vi "Playground.vi"() -> ()   [LabVIEW 2019]
uses:
  ObjectSettings/ObjectSettings.lvclass/ObjectSettings.ctl
  Setting Database/Setting Database.lvclass
  <vilib>/JKI/JKI SMO/SMO/SMO.lvclass
  Path Settings/Path Settings.lvclass
  C:/Users/Albro/Documents/GitHub/AFM-Lithography/lvsrc/Classes/Settings/ObjectSettings/ObjectSettings.lvclass
  Setting Database/Typedefs/PrivateEvents--Setting Database.CopyActivePathToAll.ctl
  <vilib>/addons/_JKI Toolkits/Caraya/classes/Test/Test.lvclass
  <vilib>/addons/_JKI Toolkits/Caraya/classes/Assert/Assert.lvclass
  <vilib>/addons/_JKI Toolkits/Caraya/classes/Assert/Assert Equal Value_Variant.vi
  ObjectSettings/ObjectSettings.lvclass
  C:/Program Files (x86)/National Instruments/LabVIEW 2019/vi.lib/JKI/JKI SMO/SMO/SMO.lvclass
  Setting Database/Typedefs/PrivateEvents--Setting Database.Refresh.ctl
panel:
  in  "Speed Settings":bool
  out "error out":errorcluster
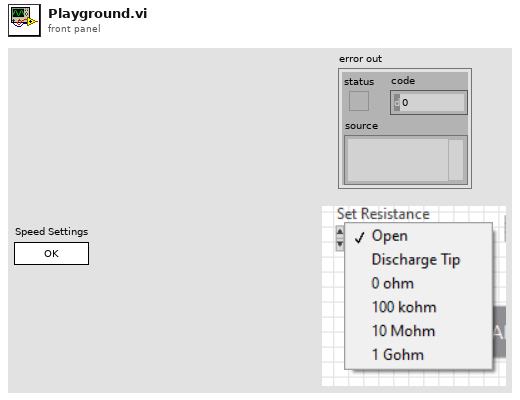
[diagram p1: front panel]
types:
  T1 = typedef "Setting Database.lvclass/PrivateEvents--Setting Database.Refresh.ctl" = cluster{"Paths":string[], "Rectangles":string[], "Funnels":string[], "Dots":string[]}
  T2 = typedef "Setting Database.lvclass/PublicEvents--Cluster.ctl" = cluster{"NewActivePath":refnum<user-event>, "PathsUpdated":refnum<user-event>, "RectanglesUpdated":refnum<user-event>, "NewActiveRectangle":refnum<user-event>, "NewActiveFunnel":refnum<user-event>, "FunnelsUpdated":refnum<user-event>, "NewActiveDot":refnum<user-event>, "DotsUpdated":refnum<user-event>}
  T3 = typedef "Setting Database.lvclass/PublicEvents--Setting Database.PathsUpdated.ctl" = refnum<class "Path Settings.lvclass">[]
  T4 = enum32{"Invalid", "Standard", "Closed", "Hidden", "Minimized", "Maximized"}
  T5 = enum32{"invalid app kind", "Development System", "Run Time System", "Student Edition", "Embedded LabVIEW", "Evaluation", "Custom"}
  T6 = typedef "Setting Database.lvclass/PrivateEvents--Setting Database.CopyActivePathToAll.ctl" = bool
  T7 = typedef "Setting Database.lvclass/PublicEvents--Setting Database.NewActivePath.ctl" = refnum<class "Path Settings.lvclass">
  T8 = cluster{"Core":cluster{"Current VI Reference":refnum<vi>, "Close Panel on Exit?":bool}, "Path Settings":refnum<class "Path Settings.lvclass">, "Your string data":string, "Setting Database":refnum<class "Setting Database.lvclass">}
  T9 = cluster{"Current VI Reference":refnum<vi>, "Close Panel on Exit?":bool}
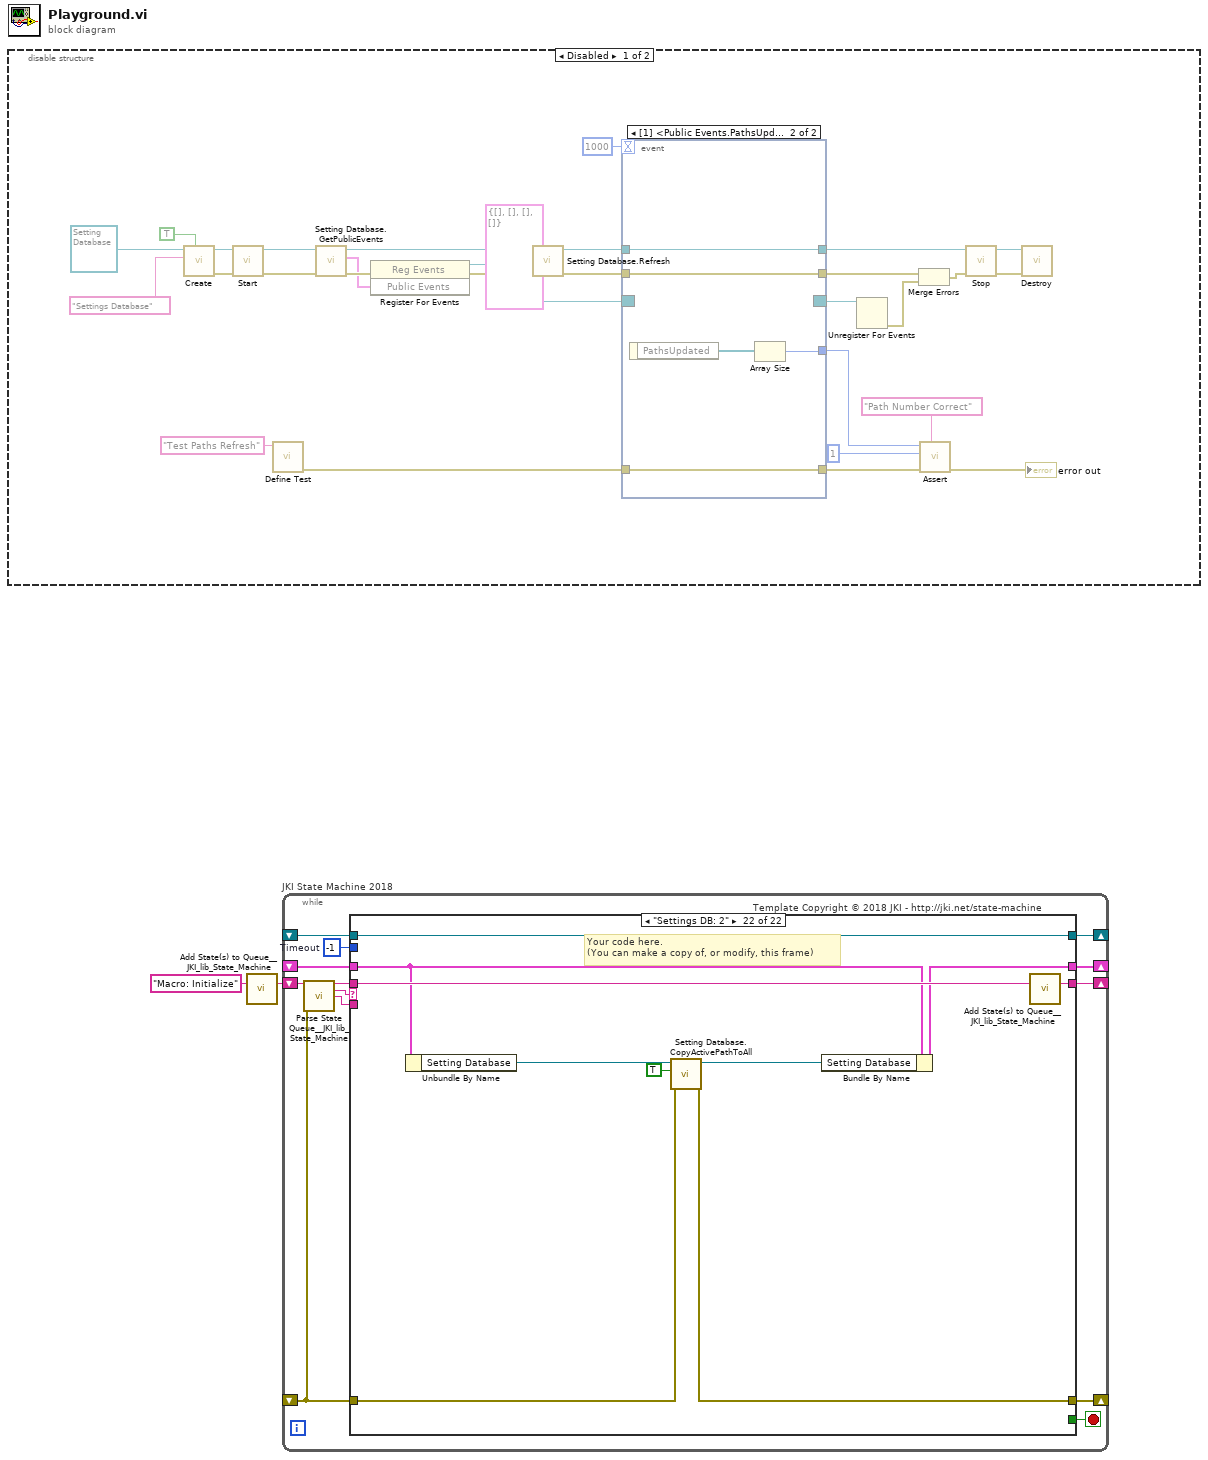
[diagram p0: block diagram]
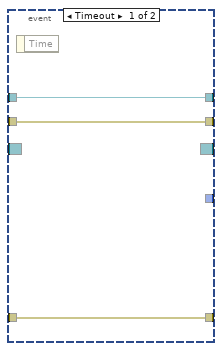
[diagram p2: hidden frame]
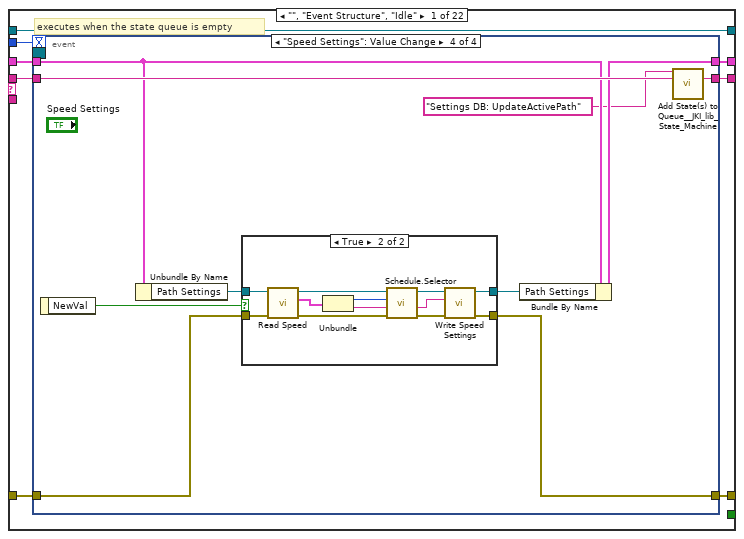
[diagram p4: hidden frame]
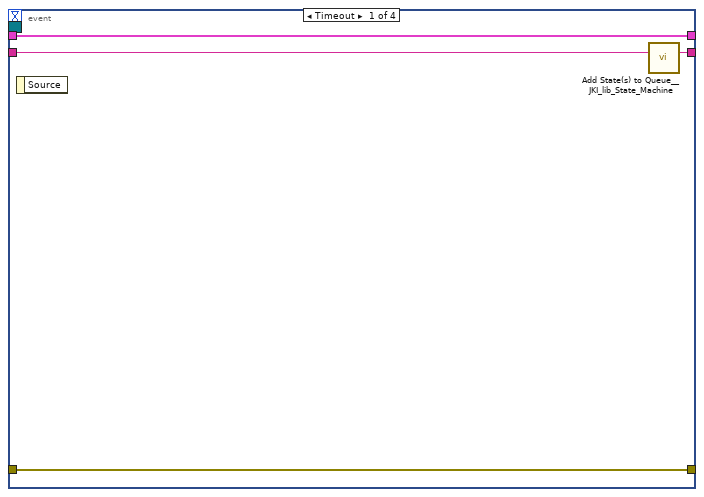
[diagram p5: hidden frame]
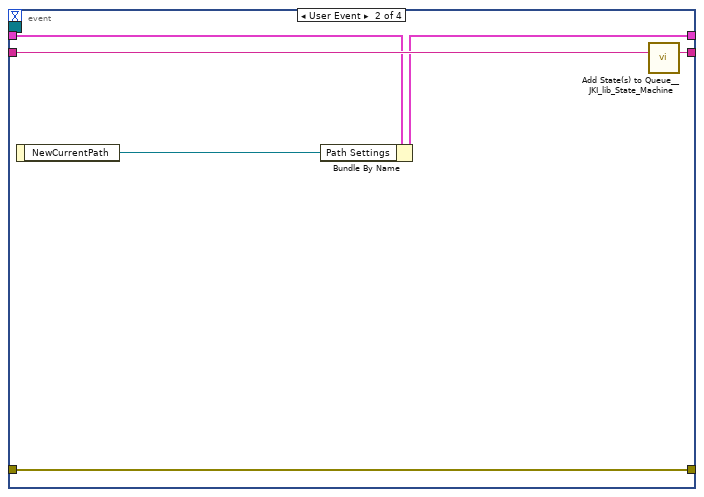
[diagram p6: hidden frame]
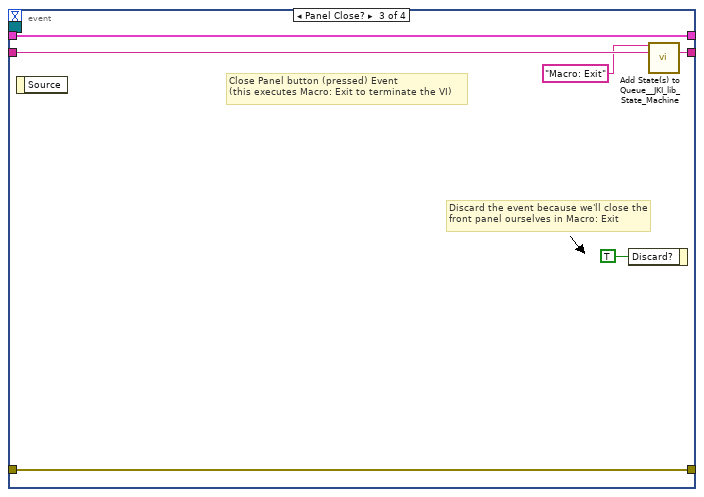
[diagram p7: hidden frame]
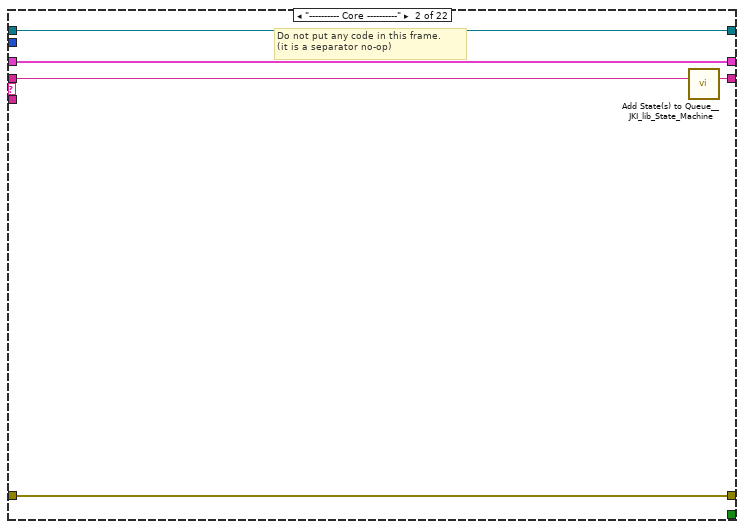
[diagram p9: hidden frame]
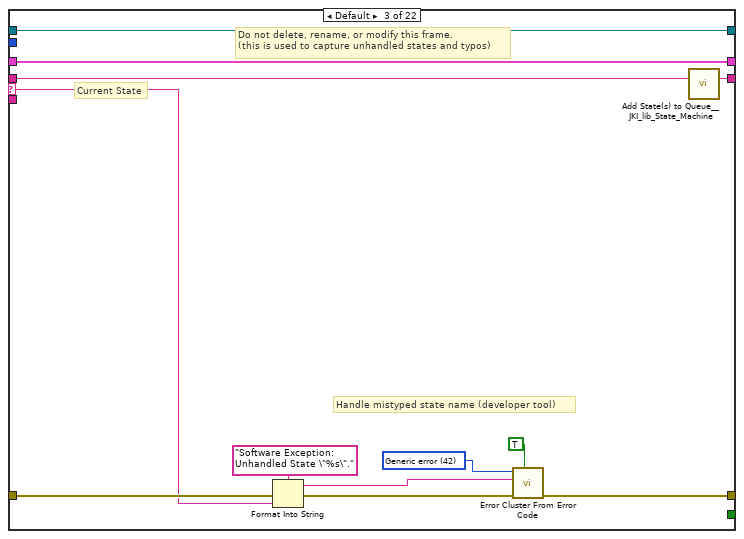
[diagram p10: hidden frame]
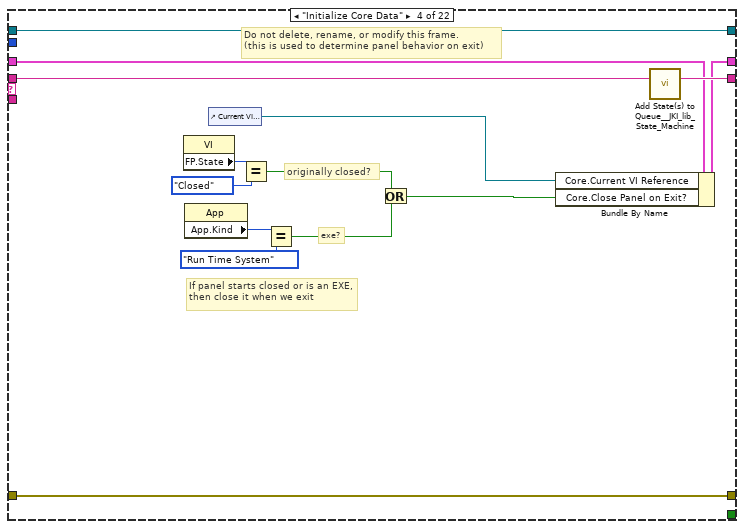
[diagram p11: hidden frame]
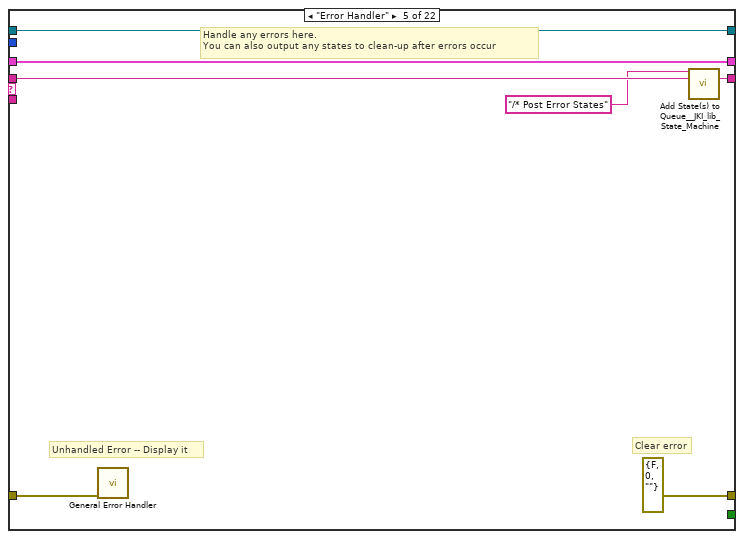
[diagram p12: hidden frame]
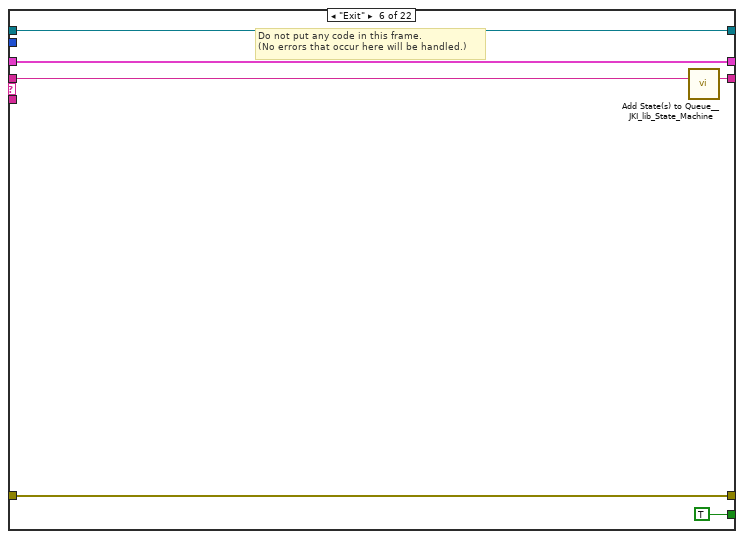
[diagram p13: hidden frame]
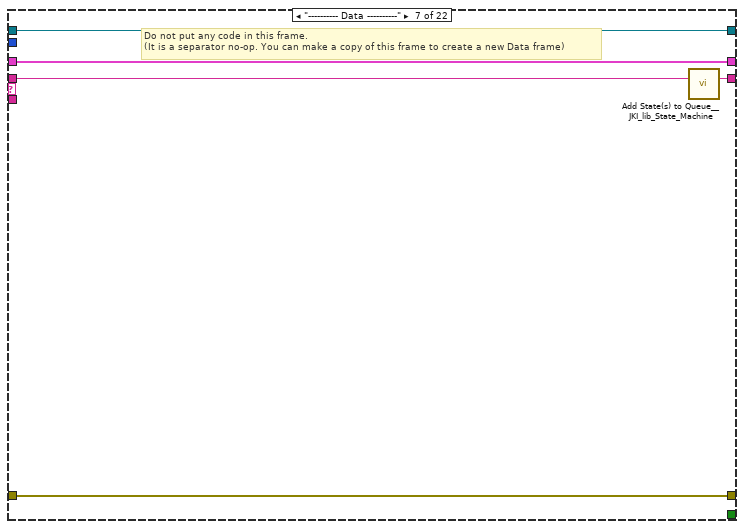
[diagram p14: hidden frame]
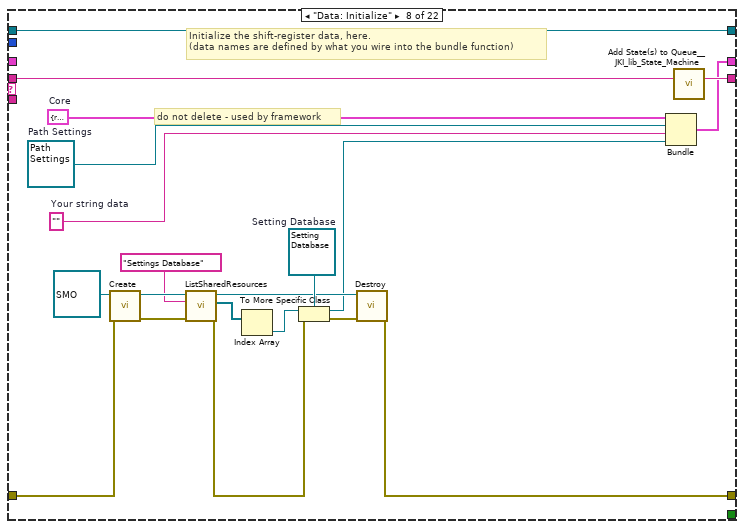
[diagram p15: hidden frame]
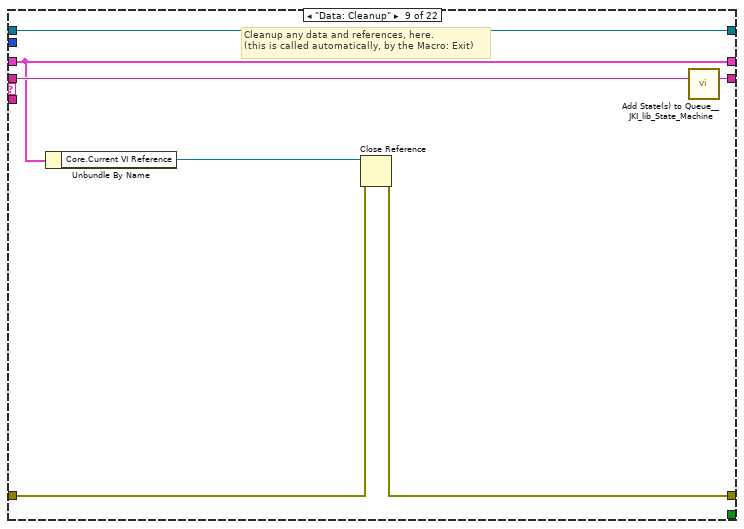
[diagram p16: hidden frame]
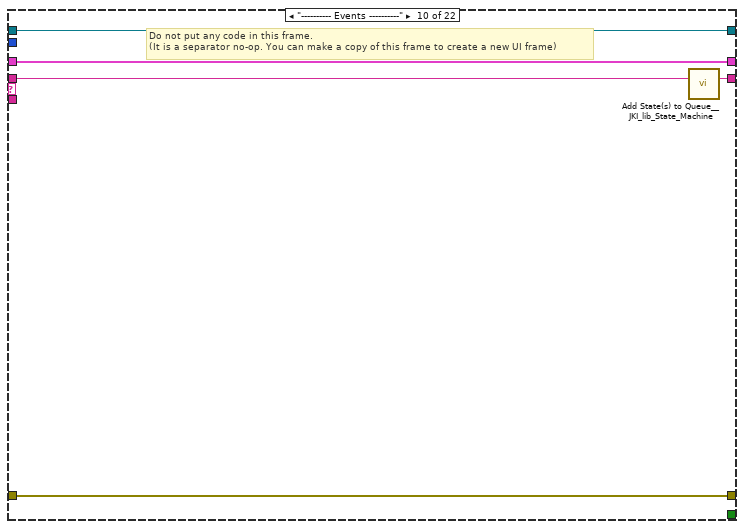
[diagram p17: hidden frame]
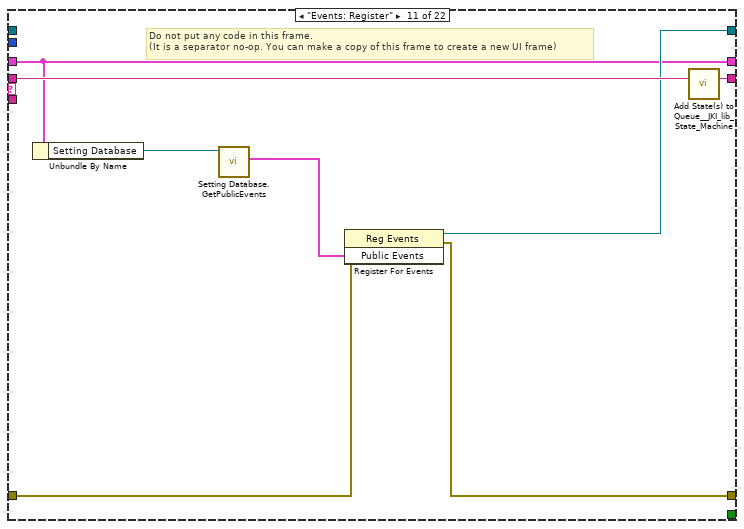
[diagram p18: hidden frame]
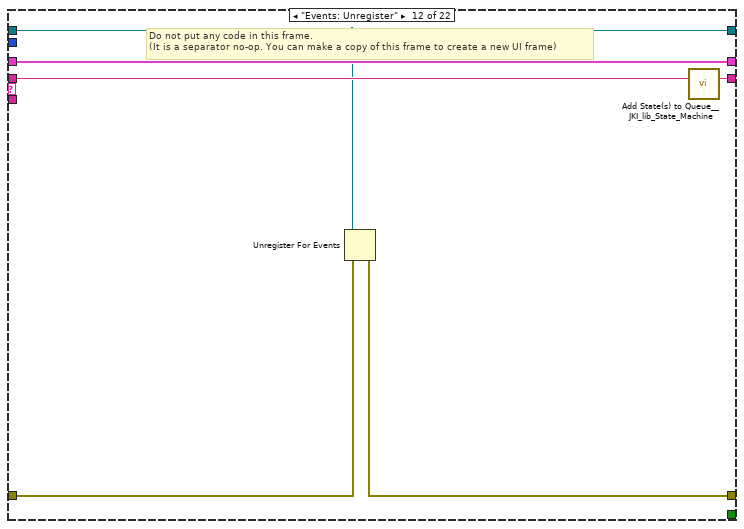
[diagram p19: hidden frame]
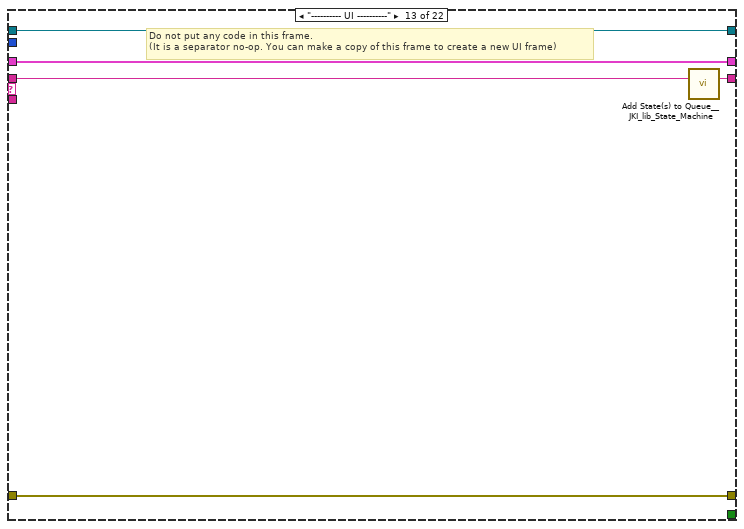
[diagram p20: hidden frame]
diagram:
  n1 = disable-structure shown="Disabled" {
    frame Disabled {
      n2 = call <vilib>:"Create.vi"("Shared Resource (F)"=TRUE, "Subsystem Name (optional)"="Settings Database", "SMO"=refnum<class "Setting Database.lvclass"> refnum ("Setting Database.lvclass")) -> ("error out"=w4:errorcluster, "SMO out"=w29:refnum<class "Setting Database.lvclass">)  [unwired: 6 in, 1 out]
      n3 = call <vilib>:"Start.vi"("error in (no error)"=w4, "SMO"=w29) -> ("error out"=w27:errorcluster, "SMO out"=w26:refnum<class "Setting Database.lvclass">)  [unwired: 8 in]
      n4 = call <vilib>:"Define Test.vi"("Label (VI Title)"="Test Paths Refresh") -> ("error out"=w11:errorcluster)  [unwired: 9 in, 1 out]
      n5 = call "Setting Database.GetPublicEvents.vi"("error in (no error)"=w27, "Setting Database"=w26) -> ("error out"=w24:errorcluster, "Public Events"=w22:T2, "Setting Database out"=w25:refnum<class "Setting Database.lvclass">)  [unwired: 7 in]
      n6 = register-events(error in=w24, w22) -> (reference out=w3:refnum<event-registration>, error out=w23:errorcluster)  [unwired: 1 in]
      n7 = call "Setting Database.Refresh.vi"("error in (no error)"=w23, "Initialize"=T1 {"Paths"=[], "Rectangles"=[], "Funnels"=[], "Dots"=[]}, "Setting Database"=w25) -> ("error out"=w17:errorcluster, "Setting Database out"=w18:refnum<class "Setting Database.lvclass">)  [unwired: 7 in]
      n8 = event shown="[1] <Public Events.PathsUpdated>: User Event" {
        selector: w3 -> [_ _]
        dyn-events: [_ _] -> w20
        timeout: 1000 -> [_ _]
        tunnel: [w35 w40] -> w19
        tunnel: w18 -> [w35 w40]
        tunnel: w17 -> [w34 w39]
        tunnel: [w34 w39] -> w16
        tunnel: [_ w37] -> w7
        tunnel: w11 -> [w33 w36]
        tunnel: [w33 w36] -> w10
        event Timeout {
          n9 = event-data() -> ()  [unwired: 1 in, 1 out]
        }
        event User Event {
          n10 = event-data() -> ("PathsUpdated"=w38:T3)  [unwired: 1 in]
          n11 = Array Size(array=w38) -> (size(s)=w37:i32)
        }
      }
      n12 = Unregister For Events(event registration refnum=w20) -> (error out=w14:errorcluster)  [unwired: 1 in]
      n13 = Merge Errors(w16, w14) -> (w15:errorcluster)
      n14 = call-poly <vilib>:"Assert.vi"("Label"="Path Number Correct", "error in (no error)"=w10, "Actual"=1 ("size(s)"), "Expected"=w7) -> ("error out"=→"error out":errorcluster)  [unwired: 6 in, 1 out]
      n15 = call <vilib>:"Stop.vi"("error in (no error)"=w15, "SMO"=w19) -> ("error out"=w13:errorcluster, "SMO out"=w28:refnum<class "Setting Database.lvclass">)  [unwired: 8 in]
      n16 = call <vilib>:"Destroy.vi"("error in (no error)"=w13, "SMO"=w28) -> ()  [unwired: 9 in, 1 out]
    }
    frame Enabled {
    }
  }
  n17 = call <vilib>:"Add State(s) to Queue__JKI_lib_State_Machine.vi"("State(s) in (\"\")"="Macro: Initialize") -> ("States Out"=w2:string)  [unwired: 14 in]
  n18 = while "JKI State Machine 2018" {
    shift-right: [w46] -> _
    shift-left: _ -> [w45]
    shift-right: [w49] -> _
    shift-left: _ -> [w43]
    shift-right: [w48] -> _
    shift-left: w2 -> [w50]
    shift-right: [w42] -> _
    shift-left: _ -> [w41]
    stop <- w47 stop-if-true
    w44 = -1  # Timeout
    # "Template Copyright © 2018 JKI - http://jki.net/state-machine"
    n19 = call <vilib>:"Parse State Queue__JKI_lib_State_Machine.vi"("State Queue"=w50, "Error In (no error)"=w43) -> ("Remaining States"=w52:string, "Current State"=w53:string, "Arguments"=w51:string)  [unwired: 11 in]
    n20 = case shown="\"Settings DB: 2\"" w53 {
      selector: w53 -> [_ _ w108 _ _ _ _ _ _ _ _ _ _ _ _ _ _ _ _ _ _ _]
      tunnel: w52 -> [w61 w106 w112 w132 w139 w145 w150 w170 w177 w182 w190 w196 w201 w206 w213 w225 w295 w301 w312 w317 w327 w337]
      tunnel: w51 -> [_ _ _ _ _ _ _ _ _ _ _ _ _ _ w208 w219 _ _ _ _ _ _]
      tunnel: w45 -> [w59 w103 w110 w125 w136 w143 w147 _ w172 w179 w186 w194 w198 w204 w211 w221 w292 w298 w309 w314 w324 w328]
      tunnel: [w58 w104 w114 w129 errorcluster {"status"=FALSE, "code"=0, "source"=""} ("error out") w142 w148 w153 w173 w180 w187 w191 w199 w203 w209 w222 w293 w299 w310 w315 w320 w334] -> w49
      tunnel: w43 -> [w57 w104 w113 w129 w135 w142 w148 w155 w174 w180 w183 w192 w199 w203 w210 w223 w293 w299 w310 w315 w319 w333]
      tunnel: [w60 w105 w111 w131 w138 w144 w149 w169 w176 w181 w189 w195 w200 w205 w212 w224 w294 w300 w311 w316 w326 w336] -> w48
      tunnel: [_ _ _ _ _ TRUE _ _ _ _ _ _ _ _ _ _ _ _ _ _ _ _] -> w47
      tunnel: [w56 w103 w110 w130 w136 w143 w147 w168 w172 w179 w186 w194 w198 w204 w211 w221 w292 w298 w309 w314 w325 w329] -> w46
      tunnel: w44 -> [w55 _ _ _ _ _ _ _ _ _ _ _ _ _ _ _ _ _ _ _ _ _]
      tunnel: [w54 w102 w107 w119 w133 w140 w146 w151 w171 w178 w188 w193 w197 w202 w207 w218 w291 w296 w302 w313 w318 w335] -> w42
      tunnel: w41 -> [w54 w102 w107 w119 w133 w140 w146 w151 w171 w178 _ w193 w197 w202 w207 w218 w291 w296 w302 w313 w318 w335]
      frame "", "Event Structure", "Idle" {
        # "executes when the state queue is empty"
        n21 = event shown="[3] \"Speed Settings\": Value Change" {
          selector: w54 -> [_ _ _ _]
          dyn-events: _ -> [_ _ _ _]
          timeout: w55 -> [_ _ _ _]
          tunnel: w61 -> [w65 w71 w77 w87]
          tunnel: [w64 w70 w76 w86] -> w60
          tunnel: w59 -> [w62 w67 w74 w79]
          tunnel: [w63 w69 w75 w80] -> w58
          tunnel: w57 -> [w63 w69 w75 w85]
          tunnel: [w62 w68 w74 w82] -> w56
          event Timeout {
            n22 = event-data() -> ()  [unwired: 1 in, 1 out]
            n23 = call <vilib>:"Add State(s) to Queue__JKI_lib_State_Machine.vi"("State(s) in (\"\")"=w65) -> ("States Out"=w64:string)  [unwired: 14 in]
          }
          event User Event {
            n24 = event-data() -> ("NewCurrentPath"=w66:T7)  [unwired: 1 in]
            n25 = Bundle By Name(cluster=w67, "Path Settings"=w66) -> (w68:T8)
            n26 = call <vilib>:"Add State(s) to Queue__JKI_lib_State_Machine.vi"("State(s) in (\"\")"=w71) -> ("States Out"=w70:string)  [unwired: 14 in]
          }
          event Panel Close? {
            # "Discard the event because we'll close the front panel ourselves in Macro: Exit"
            # "Close Panel button (pressed) Event\n(this executes Macro: Exit to terminate the VI)"
            n27 = event-data() -> ()  [unwired: 1 in, 1 out]
            n28 = event-data("Discard?"=TRUE) -> ()  [unwired: 1 in, 1 out]
            n29 = call <vilib>:"Add State(s) to Queue__JKI_lib_State_Machine.vi"("State(s) in Front (\"\")"="Macro: Exit", "State(s) in (\"\")"=w77) -> ("States Out"=w76:string)  [unwired: 13 in]
          }
          event "Speed Settings": Value Change {
            n30 = event-data() -> ("NewVal"=w81:bool)  [unwired: 1 in]
            n31 = Unbundle By Name(w79) -> ("Path Settings"=w84:refnum<class "Path Settings.lvclass">)
            n32 = case shown="True" w81 {
              tunnel: w84 -> [w89 w94]
              tunnel: [w89 w92] -> w83
              tunnel: w85 -> [w88 w91]
              tunnel: [w88 w90] -> w80
              frame False {
              }
              frame True {
                n33 = call "Read Speed.vi"("error in (no error)"=w91, "ObjectSettings in"=w94) -> ("error out"=w97:errorcluster, "Speed"=w98:cluster{"Schedule":u16, "Settings":string}, "ObjectSettings out"=w101:refnum<class "Path Settings.lvclass">)  [unwired: 7 in]
                n34 = Unbundle(w98) -> ("Schedule"=w100:u16, "Settings"=w99:string)
                n35 = call-dynamic "Schedule.Selector.vi"("error in (no error)"=w97, "Settings In"=w99, "Schedule"=w100, "ObjectSettings in"=w101) -> ("error out"=w95:errorcluster, "Settings Out"=w93:string, "ObjectSettings out"=w96:refnum<class "Path Settings.lvclass">)  [unwired: 5 in]
                n36 = call "Write Speed Settings.vi"("error in (no error)"=w95, "Settings"=w93, "ObjectSettings in"=w96) -> ("error out"=w90:errorcluster, "ObjectSettings out"=w92:refnum<class "Path Settings.lvclass">)  [unwired: 7 in]
              }
            }
            n37 = Bundle By Name(cluster=w79, "Path Settings"=w83) -> (w82:T8)
            n38 = call <vilib>:"Add State(s) to Queue__JKI_lib_State_Machine.vi"("State(s) in Front (\"\")"="Settings DB: UpdateActivePath", "State(s) in (\"\")"=w87) -> ("States Out"=w86:string)  [unwired: 13 in]
          }
        }
      }
      frame "---------- Core ----------" {
        # "Do not put any code in this frame.\n(it is a separator no-op)"
        n39 = call <vilib>:"Add State(s) to Queue__JKI_lib_State_Machine.vi"("State(s) in (\"\")"=w106) -> ("States Out"=w105:string)  [unwired: 14 in]
      }
      frame Default {
        w117 = 42 items=["No error", "Argument error", "Memory is full", "Out of zone", "End of file", "File already open", "Generic file I/O error", "File not found", "File permission error", "Disk is full", "Duplicate path", "Too many files open", "System feature not enabled", "Resource file not found", "Cannot add resource", "Resource not found", "Image not found", "Image memory error", "Pen does not exist", "Config type invalid", "Config token not found", "Config parse error", "Config memory error", "Bad external code format", "Bad external code offset", "External code not present", "Null window", "Destroy window error", "Null menu", "Print aborted", "Bad print record", "Print driver error", "Windows error during printing", "Memory error during printing", "Print dialog error", "Generic print error", "Invalid device refnum", "Device not found", "Device parameter error", "Device unit error", "Cannot open device", "Device call aborted", "Generic error", "Cancelled by user", "Object ID too low", "Object ID too high", "Object not in heap", "Unknown heap", "Unknown object (invalid DefProc)", "Unknown object (DefProc not in table)", "Message out of range", "Invalid (null) method", "Unknown message", "Manager call not supported", "Bad address", "Network operation in progress", "Network operation timed out", "Connection is busy", "Network attribute not supported", "Network error", "Address in use", "System out of memory", "Connection aborted", "Connection refused", "Not connected", "Already connected", "Connection closed", "Initialization error (interapplication manager)", "Bad occurrence", "Wait on unbound occurrence handler", "Occurrence queue overflow", "Datalog type conflict", "Unused", "Unrecognized type (interapplication manager)", "Memory corrupt", "Failed to make temporary DLL", "Old CIN version", "Drag socket not found", "Failed to load drop-object", "Failed to register OLE object", "Failed to release OLE object", "Format specifier type mismatch", "Unknown format specifier", "Too few format specifiers", "Too many format specifiers", "Scan failed", "Newer CIN version", "Error converting to variant", "Runtime menu error", "Password tampered", "Variant attribute not found", "Incompatible variant data type", "Event data is not available", "Event Store is not present", "Occurrence is not found", "Event Queue is not created", "Event info is not available", "Refnum passed is NULL", "Error retrieving Class GUID", "Error retrieving CoClass GUID", "Error retrieving TypeLib GUID.", "Bad built application magic bytes.", "Specific driver is different from the specific driver associated with the Logical Name.", "There is no session opened to the class driver.", "Max Error", "MAX - Error with config objects", "MAX - Error loading configuration", "MAX - Group not supported"]
        # "Current State"
        # "Do not delete, rename, or modify this frame.\n(this is used to capture unhandled states and typos)"
        # "Handle mistyped state name (developer tool)"
        n40 = Format Into String(format string="Software Exception: Unhandled State \"%s\"." ("message"), error in=w113, w108) -> (resulting string=w116:string, error out=w115:errorcluster)  [unwired: 1 in]
        n41 = call <vilib>:"Error Cluster From Error Code.vi"("show call chain? (False)"=TRUE, "error in (no error)"=w115, "error message (\"\")"=w116, "error code (0)"=w117) -> ("error out"=w114:errorcluster)  [unwired: 5 in]
        n42 = call <vilib>:"Add State(s) to Queue__JKI_lib_State_Machine.vi"("State(s) in (\"\")"=w112) -> ("States Out"=w111:string)  [unwired: 14 in]
      }
      frame "Initialize Core Data" {
        # "Do not delete, rename, or modify this frame.\n(this is used to determine panel behavior on exit)"
        # "originally closed?"
        # "exe?"
        # "If panel starts closed or is an EXE, then close it when we exit"
        n43 = property class="VI"() -> ("FP.State"=w122:T4)  [unwired: 2 in, 2 out]
        n44 = property class="App"() -> ("App.Kind"=w128:T5)  [unwired: 2 in, 2 out]
        n45 = control-ref of="Current VI Reference"() -> (w123:refnum<vi>)
        n46 = Equal?(x=w122, y=T4."Closed" ("Front Panel Window:State")) -> (x = y?=w120:bool)
        n47 = Equal?(x=w128, y=T5."Run Time System" ("Application:Kind")) -> (x = y?=w126:bool)
        n48 = Or(x=w120, y=w126) -> (x .or. y?=w124:bool)
        n49 = Bundle By Name(cluster=w125, "Core.Current VI Reference"=w123, "Core.Close Panel on Exit?"=w124) -> (w130:T8)
        n50 = call <vilib>:"Add State(s) to Queue__JKI_lib_State_Machine.vi"("State(s) in (\"\")"=w132) -> ("States Out"=w131:string)  [unwired: 14 in]
      }
      frame "Error Handler" {
        # "Unhandled Error -- Display it"
        # "Handle any errors here.\nYou can also output any states to clean-up after errors occur"
        # "Clear error"
        n51 = call <vilib>:"General Error Handler.vi"("error in (no error)"=w135) -> ()  [unwired: 10 in, 5 out]
        n52 = call <vilib>:"Add State(s) to Queue__JKI_lib_State_Machine.vi"("State(s) in Front (\"\")"="/* Post Error States", "State(s) in (\"\")"=w139) -> ("States Out"=w138:string)  [unwired: 13 in]
      }
      frame "Exit" {
        # "Do not put any code in this frame.\n(No errors that occur here will be handled.)"
        n53 = call <vilib>:"Add State(s) to Queue__JKI_lib_State_Machine.vi"("State(s) in (\"\")"=w145) -> ("States Out"=w144:string)  [unwired: 14 in]
      }
      frame "---------- Data ----------" {
        # "Do not put any code in this frame.\n(It is a separator no-op. You can make a copy of this frame to create a new Data frame)"
        n54 = call <vilib>:"Add State(s) to Queue__JKI_lib_State_Machine.vi"("State(s) in (\"\")"=w150) -> ("States Out"=w149:string)  [unwired: 14 in]
      }
      frame "Data: Initialize" {
        w152 = refnum<class "Path Settings.lvclass"> refnum  # Path Settings
        w161 = refnum<class "Setting Database.lvclass"> refnum  # Setting Database
        w167 = T9 {"Current VI Reference"=refnum, "Close Panel on Exit?"=FALSE}  # Core
        w166 = ""  # Your string data
        # "do not delete - used by framework"
        # "Initialize the shift-register data, here.\n(data names are defined by what you wire into the bundle function)"
        n55 = call <vilib>:"Create.vi"("error in (no error)"=w155, "SMO"=refnum<class "SMO.lvclass"> refnum) -> ("error out"=w157:errorcluster, "SMO out"=w165:refnum<class "SMO.lvclass">)  [unwired: 7 in, 1 out]
        n56 = call <vilib>:"ListSharedResources.vi"("error in (no error)"=w157, "Filter (regex|name)"="Settings Database" ("Subsystem Name (optional)"), "SMO in"=w165) -> ("error out"=w154:errorcluster, "Shared Resources"=w163:refnum<class "SMO.lvclass">[], "SMO out"=w159:refnum<class "SMO.lvclass">)  [unwired: 5 in, 1 out]
        n57 = Index Array(array=w163) -> (element=w162:refnum<class "SMO.lvclass">)  [unwired: 1 in]
        n58 = To More Specific Class(target class=w161, reference=w162, error in=w154) -> (specific class reference=w156:refnum<class "Setting Database.lvclass">, error out=w158:errorcluster)
        n59 = call <vilib>:"Destroy.vi"("error in (no error)"=w158, "SMO"=w159) -> ("error out"=w153:errorcluster)  [unwired: 9 in]
        n60 = Bundle("Core"=w167, "Path Settings"=w152, "Your string data"=w166, "Setting Database"=w156) -> (w168:T8)  [unwired: 1 in]
        n61 = call <vilib>:"Add State(s) to Queue__JKI_lib_State_Machine.vi"("State(s) in (\"\")"=w170) -> ("States Out"=w169:string)  [unwired: 14 in]
      }
      frame "Data: Cleanup" {
        # "Cleanup any data and references, here.\n(this is called automatically, by the Macro: Exit)"
        n62 = Unbundle By Name(w172) -> ("Core.Current VI Reference"=w175:refnum<vi>)
        n63 = Close Reference(reference=w175, error in (no error)=w174) -> (error out=w173:errorcluster)
        n64 = call <vilib>:"Add State(s) to Queue__JKI_lib_State_Machine.vi"("State(s) in (\"\")"=w177) -> ("States Out"=w176:string)  [unwired: 14 in]
      }
      frame "---------- Events ----------" {
        # "Do not put any code in this frame.\n(It is a separator no-op. You can make a copy of this frame to create a new UI frame)"
        n65 = call <vilib>:"Add State(s) to Queue__JKI_lib_State_Machine.vi"("State(s) in (\"\")"=w182) -> ("States Out"=w181:string)  [unwired: 14 in]
      }
      frame "Events: Register" {
        # "Do not put any code in this frame.\n(It is a separator no-op. You can make a copy of this frame to create a new UI frame)"
        n66 = Unbundle By Name(w186) -> ("Setting Database"=w185:refnum<class "Setting Database.lvclass">)
        n67 = call "Setting Database.GetPublicEvents.vi"("Setting Database"=w185) -> ("Public Events"=w184:T2)  [unwired: 8 in, 2 out]
        n68 = register-events(error in=w183, w184) -> (reference out=w188:refnum<event-registration>, error out=w187:errorcluster)  [unwired: 1 in]
        n69 = call <vilib>:"Add State(s) to Queue__JKI_lib_State_Machine.vi"("State(s) in (\"\")"=w190) -> ("States Out"=w189:string)  [unwired: 14 in]
      }
      frame "Events: Unregister" {
        # "Do not put any code in this frame.\n(It is a separator no-op. You can make a copy of this frame to create a new UI frame)"
        n70 = Unregister For Events(event registration refnum=w193, error in=w192) -> (error out=w191:errorcluster)
        n71 = call <vilib>:"Add State(s) to Queue__JKI_lib_State_Machine.vi"("State(s) in (\"\")"=w196) -> ("States Out"=w195:string)  [unwired: 14 in]
      }
      frame "---------- UI ----------" {
        # "Do not put any code in this frame.\n(It is a separator no-op. You can make a copy of this frame to create a new UI frame)"
        n72 = call <vilib>:"Add State(s) to Queue__JKI_lib_State_Machine.vi"("State(s) in (\"\")"=w201) -> ("States Out"=w200:string)  [unwired: 14 in]
      }
      frame "UI: Initialize" {
        # "Initialize the User Interface, here.\n(this is called automatically, by the Macro: Init)"
        n73 = call <vilib>:"Add State(s) to Queue__JKI_lib_State_Machine.vi"("State(s) in (\"\")"=w206) -> ("States Out"=w205:string)  [unwired: 14 in]
      }
      frame "UI: Cursor Set" {
        # "Argument"
        # "Set and Unset Cursor Busy.\n(Usage: \"UI: Cursor Set >> Busy|Idle\")"
        n74 = case shown="\"Idle\", Default" w208 {
          tunnel: w210 -> [w215 w217]
          tunnel: [w214 w216] -> w209
          frame "Idle", Default {
            n75 = call <vilib>:"Unset Busy.vi"("error in (no error)"=w215) -> ("error out"=w214:errorcluster)  [unwired: 10 in]
          }
          frame "Busy" {
            n76 = call <vilib>:"Set Busy.vi"("error in (no error)"=w217) -> ("error out"=w216:errorcluster)  [unwired: 9 in, 1 out]
          }
        }
        n77 = call <vilib>:"Add State(s) to Queue__JKI_lib_State_Machine.vi"("State(s) in (\"\")"=w213) -> ("States Out"=w212:string)  [unwired: 14 in]
      }
      frame "UI: Front Panel State" {
        # "Argument"
        # "Set Front Panel Open or Closed\n(Usage: \"UI: Front Panel State >> Open|Close\")"
        n78 = Unbundle By Name(w221) -> ("Core.Current VI Reference"=w220:refnum<vi>)
        n79 = case shown="\"Minimize\", \"Minimized\"" w219 {
          tunnel: w223 -> [w231 w246 w257 w270 w283]
          tunnel: [w233 w247 w259 w272 w285] -> w222
          tunnel: w220 -> [w232 w244 w258 w271 w284]
          frame "Open", "Standard", Default {
            w226 = T4."Standard" ("State")
            n80 = property class="VI"(reference=w232, error in=w231) -> (reference out=w229:refnum<vi>, error out=w230:errorcluster, "FP.State"=w228:T4)
            n81 = Not Equal?(x=w228, y=w226) -> (x != y?=w227:bool)
            n82 = case shown="True" w227 {
              tunnel: [w237 w239] -> w233
              tunnel: w230 -> [w236 w239]
              tunnel: w229 -> [w235 _]
              tunnel: w226 -> [w234 _]
              frame True {
                n83 = invoke class="VI" method="FP.Open"(reference=w235, error in=w236, "Activate"=TRUE, "State"=w234) -> (error out=w237:errorcluster)  [unwired: 1 in, 4 out]
              }
              frame False {
              }
            }
          }
          frame "Close", "Closed" {
            n84 = property class="VI"(reference=w244, error in=w246) -> (reference out=w243:refnum<vi>, error out=w245:errorcluster, "FP.State"=w241:T4)
            n85 = Not Equal?(x=w241, y=T4."Closed" ("Front Panel Window:State")) -> (x != y?=w240:bool)
            n86 = case shown="True" w240 {
              tunnel: [w248 w251] -> w247
              tunnel: w245 -> [w248 w250]
              tunnel: w243 -> [_ w249]
              frame False {
              }
              frame True {
                n87 = invoke class="VI" method="FP.Close"(reference=w249, error in=w250) -> (error out=w251:errorcluster)  [unwired: 1 in, 2 out]
              }
            }
          }
          frame "Hidden", "Hide" {
            w252 = T4."Hidden" ("State")
            n88 = property class="VI"(reference=w258, error in=w257) -> (reference out=w255:refnum<vi>, error out=w256:errorcluster, "FP.State"=w254:T4)
            n89 = Not Equal?(x=w254, y=w252) -> (x != y?=w253:bool)
            n90 = case shown="True" w253 {
              tunnel: [w263 w264] -> w259
              tunnel: w256 -> [w262 w264]
              tunnel: w255 -> [w261 _]
              tunnel: w252 -> [w260 _]
              frame True {
                n91 = invoke class="VI" method="FP.Open"(reference=w261, error in=w262, "State"=w260) -> (error out=w263:errorcluster)  [unwired: 2 in, 4 out]
              }
              frame False {
              }
            }
          }
          frame "Minimize", "Minimized" {
            w265 = T4."Minimized" ("State")
            n92 = property class="VI"(reference=w271, error in=w270) -> (reference out=w268:refnum<vi>, error out=w269:errorcluster, "FP.State"=w267:T4)
            n93 = Not Equal?(x=w267, y=w265) -> (x != y?=w266:bool)
            n94 = case shown="True" w266 {
              tunnel: [w276 w277] -> w272
              tunnel: w269 -> [w275 w277]
              tunnel: w268 -> [w274 _]
              tunnel: w265 -> [w273 _]
              frame True {
                n95 = invoke class="VI" method="FP.Open"(reference=w274, error in=w275, "State"=w273) -> (error out=w276:errorcluster)  [unwired: 2 in, 4 out]
              }
              frame False {
              }
            }
          }
          frame "Maximize", "Maximized" {
            w278 = T4."Maximized" ("State")
            n96 = property class="VI"(reference=w284, error in=w283) -> (reference out=w281:refnum<vi>, error out=w282:errorcluster, "FP.State"=w280:T4)
            n97 = Not Equal?(x=w280, y=w278) -> (x != y?=w279:bool)
            n98 = case shown="True" w279 {
              tunnel: [w289 w290] -> w285
              tunnel: w282 -> [w288 w290]
              tunnel: w281 -> [w287 _]
              tunnel: w278 -> [w286 _]
              frame True {
                n99 = invoke class="VI" method="FP.Open"(reference=w287, error in=w288, "State"=w286) -> (error out=w289:errorcluster)  [unwired: 2 in, 4 out]
              }
              frame False {
              }
            }
          }
        }
        n100 = call <vilib>:"Add State(s) to Queue__JKI_lib_State_Machine.vi"("State(s) in (\"\")"=w225) -> ("States Out"=w224:string)  [unwired: 14 in]
      }
      frame "---------- Macro ----------" {
        # "Do not put any code in this frame.\n(It is a separator no-op. You can make a copy of this frame to create a new Macro frame)"
        n101 = call <vilib>:"Add State(s) to Queue__JKI_lib_State_Machine.vi"("State(s) in (\"\")"=w295) -> ("States Out"=w294:string)  [unwired: 14 in]
      }
      frame "Macro: Initialize" {
        # "Initialization Macro\n(This is called once, when the VI starts)"
        n102 = call <vilib>:"Add State(s) to Queue__JKI_lib_State_Machine.vi"("State(s) in Front (\"\")"="Data: Initialize\nInitialize Core Data\nEvents: Register\nUI: Initialize\nUI: Front Panel State >> Open", "State(s) in (\"\")"=w301) -> ("States Out"=w300:string)  [unwired: 13 in]
      }
      frame "Macro: Exit" {
        # "Exit Macro\n(This is called once, when the VI exits)"
        n103 = Unbundle By Name(w309) -> ("Core.Close Panel on Exit?"=w308:bool)
        n104 = Select(t="UI: Front Panel State >> Close", s=w308, f="") -> (s? t:f=w305:string)
        n105 = call <vilib>:"Add State(s) to Queue__JKI_lib_State_Machine.vi"("State(s) in (\"\")"=w305, "State(s) at Back (\"\")"="Data: Cleanup\nEvents: Unregister\nExit") -> ("States Out"=w303:string)  [unwired: 13 in]
        n106 = call <vilib>:"Add State(s) to Queue__JKI_lib_State_Machine.vi"("State(s) in Front (\"\")"=w303, "State(s) in (\"\")"=w312) -> ("States Out"=w311:string)  [unwired: 13 in]
      }
      frame "---------- Settings DB ----------" {
        # "Template Separator\n(You can make a copy of, or modify, this frame)"
        n107 = call <vilib>:"Add State(s) to Queue__JKI_lib_State_Machine.vi"("State(s) in (\"\")"=w317) -> ("States Out"=w316:string)  [unwired: 14 in]
      }
      frame "Settings DB: UpdateActivePath" {
        # "Your code here.\n(You can make a copy of, or modify, this frame)"
        n108 = Unbundle By Name(w324) -> ("Setting Database"=w323:refnum<class "Setting Database.lvclass">, "Path Settings"=w321:refnum<class "Path Settings.lvclass">)
        n109 = call "Setting Database.UpdateActivePath.vi"("error in (no error)"=w319, "UpdateCurrentPath"=w321, "Setting Database"=w323) -> ("error out"=w320:errorcluster, "Setting Database"=w322:refnum<class "Setting Database.lvclass">)  [unwired: 7 in]
        n110 = Bundle By Name(cluster=w324, "Setting Database"=w322) -> (w325:T8)
        n111 = call <vilib>:"Add State(s) to Queue__JKI_lib_State_Machine.vi"("State(s) in (\"\")"=w327) -> ("States Out"=w326:string)  [unwired: 14 in]
      }
      frame "Settings DB: 2" {
        # "Your code here.\n(You can make a copy of, or modify, this frame)"
        n112 = Unbundle By Name(w328) -> ("Setting Database"=w332:refnum<class "Setting Database.lvclass">)
        n113 = call "Setting Database.CopyActivePathToAll.vi"("error in (no error)"=w333, "CopyActiveToAll"=T6 TRUE, "Setting Database"=w332) -> ("error out"=w334:errorcluster, "Setting Database out"=w330:refnum<class "Setting Database.lvclass">)  [unwired: 7 in]
        n114 = Bundle By Name(cluster=w328, "Setting Database"=w330) -> (w329:T8)
        n115 = call <vilib>:"Add State(s) to Queue__JKI_lib_State_Machine.vi"("State(s) in (\"\")"=w337) -> ("States Out"=w336:string)  [unwired: 14 in]
      }
    }
  }
